vi "Query Range Test.vi"(8 "error in (no error)":errorcluster {"code" format="%.0x"}, 11 "VISA resource name":refnum<visa-resource-name>) -> (0 "error out":errorcluster {"code" format="%.0x"}, 2 "Out of Range":bool, 3 "VISA resource name out":refnum<visa-resource-name>)   [LabVIEW 2015, in "Template - Power Meter.lvlib"]
doc: "Queries the instrument to determine if the upper or lower limit has been exceeded. The properties of the range can be configured by calling the <b>Configure Range</b> VI."
uses:
  <instrlib>/_Template - Power Meter/Template - Power Meter.lvlib
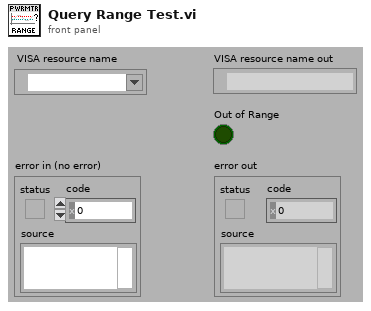
[diagram p1: front panel]
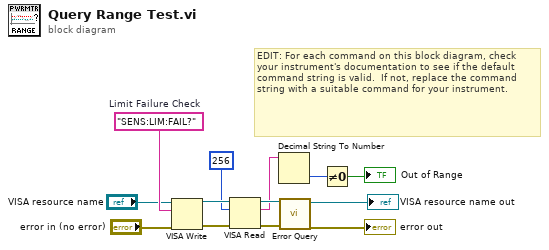
[diagram p0: block diagram]
diagram:
  w4 = "SENS:LIM:FAIL?"  # Limit Failure Check
  # "EDIT: For each command on this block diagram, check your instrument's documentation to see if the default command string is valid.  If not, replace the command string with a suitable command for your instrument."
  n1 = VISA Write(VISA resource name="VISA resource name", write buffer=w4, error in (no error)="error in (no error)") -> (VISA resource name out=w8:refnum<visa-resource-name>, error out=w9:errorcluster)  [unwired: 1 out]
  n2 = VISA Read(VISA resource name=w8, byte count=u32 256, error in (no error)=w9) -> (VISA resource name out=w10:refnum<visa-resource-name>, read buffer=w5:string, error out=w11:errorcluster)  [unwired: 1 out]
  n3 = Decimal String To Number(string=w5) -> (number=w7:i32)  [unwired: 2 in, 1 out]
  n4 = call <instrlib>:"Error Query.vi"("error in (no error)"=w11, "VISA resource name"=w10) -> ("error out"=→"error out":errorcluster, "VISA resource name out"=→"VISA resource name out":refnum<visa-resource-name>)  [unwired: 6 in, 2 out]
  n5 = Not Equal To 0?(x=w7) -> (x != 0?=→"Out of Range":bool)
